vi "3_2.vi"() -> ()   [LabVIEW 2018]
uses:
  D:/LABVIEW/examples/Instrument IO/Serial/support/Serial - Settings.ctl
  D:/LABVIEW/examples/Instrument IO/Serial/support/Serial - XON-XOFF Characters.ctl
  D:/LABVIEW/examples/Instrument IO/Serial/support/Serial - ASCII Characters.ctl
  <vilib>/Instr/_visa.llb/VISA Configure Serial Port (Instr).vi
panel:
  out "返回的字符串":string
  out "返回数据做的波形":i32[](graph)
  out "接收的数据":string
  out "布尔 3":bool
  in  "XON/XOFF校验字符":T1={"XON"=enum."DC1", "XOFF"=enum."DC3"}
  in  "停止采集":bool
  in  "开始采集":bool
  in  "串口设置":T3={"波特率"=9600, "数据位"=8, "校验"=enum."None", "停止位"=10, "流控制"=0} {"流控制" items=["无"=0, "XON/XOFF"=1, "RTS/CTS"=2, "DTR/DSR"=4]; "停止位" items=["1.0"=10, "1.5"=15, "2.0"=20]; "数据位" min=5 max=8 step=1; "波特率" items=["75"=75, "110"=110, "134"=134, "150"=150, "300"=300, "600"=600, "1200"=1200, "1800"=1800, "2400"=2400, "4800"=4800, "7200"=7200, "9600"=9600, "14400"=14400, "19200"=19200, "28800"=28800, "38400"=38400, "56000"=56000, "57600"=57600, "115200"=115200, "128000"=128000, "230400"=230400]}
  in  "串口资源":refnum<visa-resource-name>="COM1"
  in  "停止":bool
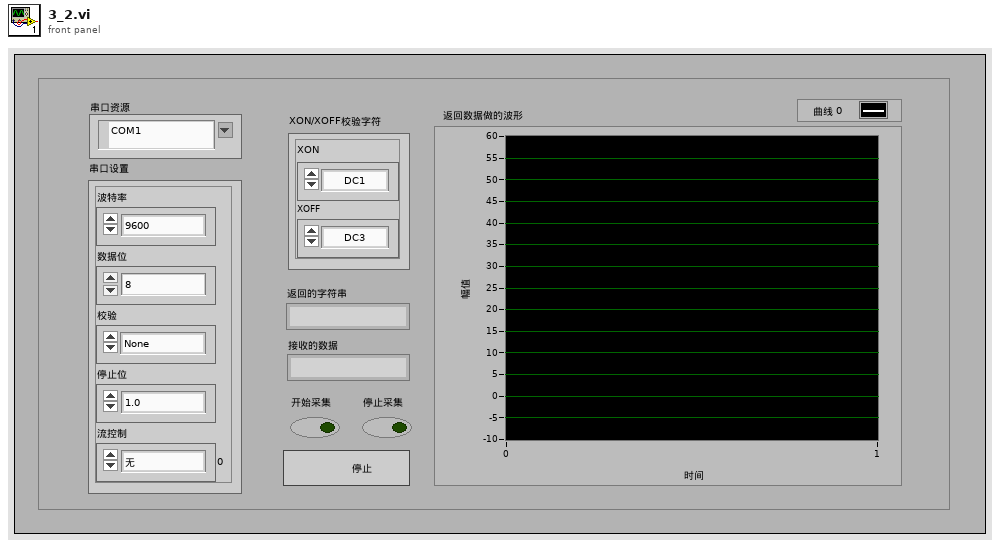
[diagram p1: front panel]
types:
  T1 = typedef "Serial - XON-XOFF Characters.ctl" = cluster{"XON":T2, "XOFF":T2}
  T2 = typedef "Serial - ASCII Characters.ctl" = enum16{"NUL", "SOH", "STX", "ETX", "EOT", "ENQ", "ACK", "BEL", "BS", "HT", "LF", "VT", "FF", "CR", "SO", "SI", "DLE", "DC1", "DC2", "DC3", "DC4", "NAK", "SYN", "ETB", "CAN", "EM", "SUB", "ESC", "FS", "GS", "RS", "US", "SP", "!", "\"", "#", "$", "%", "&", "'", "(", ")", "*", "+", ",", "- (-)", ".", "/", "0", "1", "2", "3", "4", "5", "6", "7", "8", "9", ":", ";", "<", "=", ">", "?", "@", "A", "B", "C", "D", "E", "F", "G", "H", "I", "J", "K", "L", "M", "N", "O", "P", "Q", "R", "S", "T", "U", "V", "W", "X", "Y", "Z", "[", "\\", "]", "^", "_", "`", "a", "b", "c", "d", "e", "f", "g", "h", "i", "j", "k", "l", "m", "n", "o", "p", "q", "r", "s", "t", "u", "v", "w", "x", "y", "z", "{", "|", "}", "~"}
  T3 = typedef "Serial - Settings.ctl" = cluster{"波特率":u32, "数据位":u16, "校验":enum16{"None", "Odd", "Even", "Mark", "Space"}, "停止位":u16, "流控制":u16}
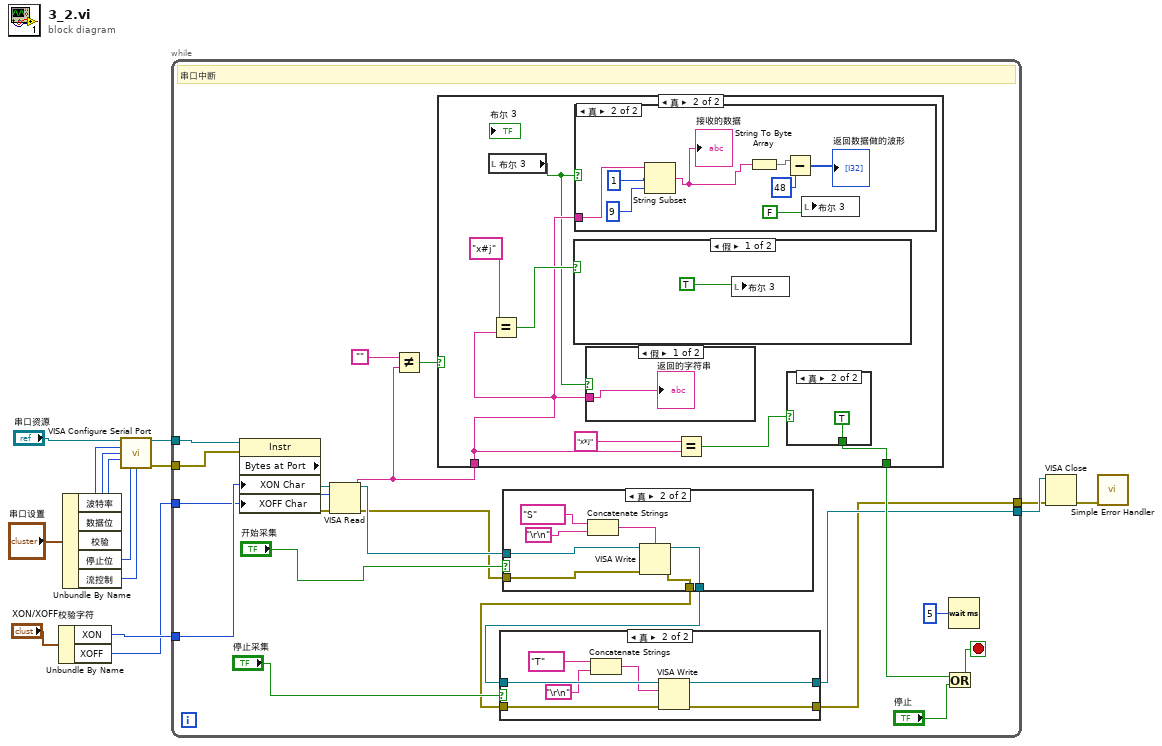
[diagram p0: block diagram]
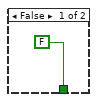
[diagram p4: hidden frame]
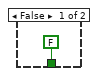
[diagram p7: hidden frame]
diagram:
  n1 = Unbundle By Name("XON/XOFF校验字符") -> ("XON"=w4:T2, "XOFF"=w3:T2)
  n2 = Unbundle By Name("串口设置") -> ("波特率"=w13:u32, "数据位"=w12:u16, "校验"=w11:enum16{"None", "Odd", "Even", "Mark", "Space"}, "停止位"=w10:u16, "流控制"=w9:u16)
  n3 = call-poly "VISA Configure Serial Port"("VISA resource name"="串口资源", "baud rate (9600)"=w13, "data bits (8)"=w12, "parity (0:none)"=w11, "stop bits (10: 1 bit)"=w10, "flow control (0:none)"=w9) -> ("VISA resource name out"=w7:refnum<visa-resource-name>, "error out"=w8:errorcluster)  [unwired: 3 in, 5 out]
  n4 = while {
    tunnel: w7 -> [w27]
    tunnel: w8 -> [w26]
    tunnel: w4 -> [w19]
    tunnel: w3 -> [w18]
    tunnel: [w17] -> w2
    tunnel: [w16] -> w1
    stop <- w30 stop-if-true
    # "串口中断"
    n5 = property class="Instr"(reference=w27, error in=w26, "XON Char"=w19, "XOFF Char"=w18) -> (reference out=w35:refnum<visa-resource-name>, error out=w34:errorcluster, "Bytes at Port"=w36:u32)
    n6 = VISA Read(VISA resource name=w35, byte count=w36, error in (no error)=w34) -> (VISA resource name out=w23:refnum<visa-resource-name>, read buffer=w32:string, error out=w22:errorcluster)  [unwired: 1 out]
    n7 = Not Equal?(x="", y=w32) -> (x != y?=w31:bool)
    n8 = case shown="真" w31 {
      tunnel: w32 -> [_ w58]
      tunnel: [FALSE w62] -> w28
      frame False {
      }
      frame True {
        n9 = local read "布尔 3"() -> (w57:bool)
        n10 = Equal?(x="x#j", y=w58) -> (x = y?=w59:bool)
        n11 = case shown="假" w59 {
          frame False {
            n12 = local write "布尔 3"(TRUE) -> ()
          }
          frame True {
          }
        }
        n13 = case shown="真" w57 {
          tunnel: w58 -> [_ w71]
          frame False {
          }
          frame True {
            n14 = String Subset(string=w71, offset (0)=1, length (rest)=9) -> (substring=w68:string)
            "接收的数据" <- w68
            n15 = String To Byte Array(string=w68) -> (unsigned byte array=w66:u8[])
            n16 = Subtract(x=w66, y=48) -> (x-y=→"返回数据做的波形":i32[])
            n17 = local write "布尔 3"(FALSE) -> ()
          }
        }
        n18 = case shown="假" w57 {
          tunnel: w58 -> [w64 _]
          frame False {
            "返回的字符串" <- w64
          }
          frame True {
          }
        }
        n19 = Equal?(x="x*j", y=w58) -> (x = y?=w61:bool)
        n20 = case shown="真" w61 {
          tunnel: [FALSE TRUE] -> w62
          frame False {
          }
          frame True {
          }
        }
      }
    }
    n21 = case shown="真" "开始采集" {
      tunnel: w23 -> [w48 w55]
      tunnel: w22 -> [w47 w54]
      tunnel: [w48 w53] -> w21
      tunnel: [w47 w52] -> w20
      frame False {
      }
      frame True {
        n22 = Concatenate Strings("S", "\r\n") -> (w51:string)
        n23 = VISA Write(VISA resource name=w55, write buffer=w51, error in (no error)=w54) -> (VISA resource name out=w53:refnum<visa-resource-name>, error out=w52:errorcluster)  [unwired: 1 out]
      }
    }
    n24 = case shown="真" "停止采集" {
      tunnel: w21 -> [w39 w46]
      tunnel: w20 -> [w38 w45]
      tunnel: [w39 w44] -> w17
      tunnel: [w38 w43] -> w16
      frame False {
      }
      frame True {
        n25 = Concatenate Strings("T", "\r\n") -> (w40:string)
        n26 = VISA Write(VISA resource name=w46, write buffer=w40, error in (no error)=w45) -> (VISA resource name out=w44:refnum<visa-resource-name>, error out=w43:errorcluster)  [unwired: 1 out]
      }
    }
    n27 = Or(x=w28, y="停止") -> (x .or. y?=w30:bool)
    n28 = Wait (ms)(milliseconds to wait=u32 5) -> ()  [unwired: 1 out]
  }
  n29 = VISA Close(VISA resource name=w2, error in (no error)=w1) -> (error out=w6:errorcluster)
  n30 = call <vilib>:"Simple Error Handler.vi"("error in (no error)"=w6) -> ()  [unwired: 1 in, 8 out]
